vi "DIY Four Flipping Coins (Cueva).vi"() -> ()   [LabVIEW 2014]
uses:
  <vilib>/Analysis/NI_AALBase.lvlib
panel:
  out "Waveform Graph":i32[](graph)
  in  "Total Number of Trials":dbl
  out "Number of Heads":i32
  out "Coin 4":bool
  out "Coin 3":bool
  out "Coin 2":bool
  out "Coin 1":bool
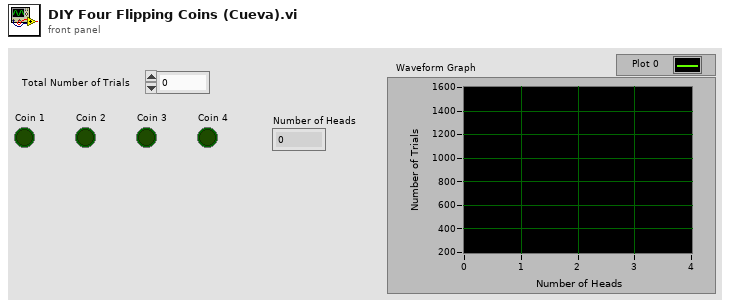
[diagram p1: front panel]
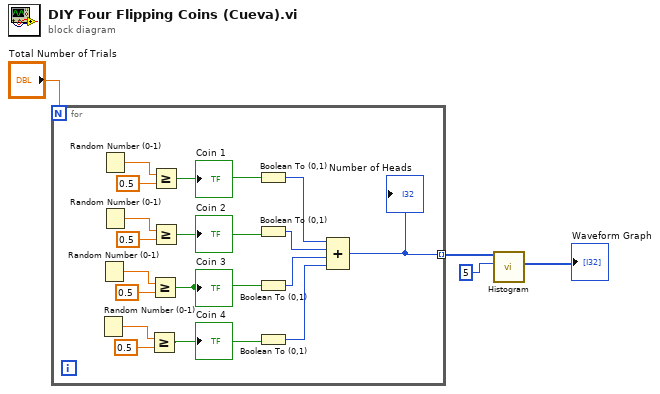
[diagram p0: block diagram]
diagram:
  n1 = for {
    N: "Total Number of Trials" -> [_]
    tunnel: [w5] -> w3 mode=indexing
    n2 = Random Number (0-1)() -> (number: 0 to 1=w15:dbl)
    n3 = Random Number (0-1)() -> (number: 0 to 1=w16:dbl)
    n4 = Random Number (0-1)() -> (number: 0 to 1=w20:dbl)
    n5 = Random Number (0-1)() -> (number: 0 to 1=w19:dbl)
    n6 = Greater Or Equal?(x=w15, y=0.5) -> (x >= y?=w12:bool)
    "Coin 4" <- w12
    n7 = Greater Or Equal?(x=w16, y=0.5) -> (x >= y?=w11:bool)
    "Coin 3" <- w11
    n8 = Greater Or Equal?(x=w20, y=0.5) -> (x >= y?=w13:bool)
    "Coin 1" <- w13
    n9 = Greater Or Equal?(x=w19, y=0.5) -> (x >= y?=w10:bool)
    "Coin 2" <- w10
    n10 = Boolean To (0,1)(Boolean=w13) -> (0, 1=w9:i16)
    n11 = Boolean To (0,1)(Boolean=w10) -> (0, 1=w8:i16)
    n12 = Boolean To (0,1)(Boolean=w11) -> (0, 1=w7:i16)
    n13 = Boolean To (0,1)(Boolean=w12) -> (0, 1=w6:i16)
    n14 = Compound Arithmetic op=ADD(w9, w8, w7, w6) -> (w5:i16)
    "Number of Heads" <- w5
  }
  n15 = call <vilib>:"Histogram.vi"("intervals"=5, "X"=w3) -> ("Histogram: h(x)"=→"Waveform Graph":i32[])  [unwired: 6 in, 3 out]
